vi "LockinDAQ.Write AO.vi"(8 "error in (no error)":errorcluster, 10 "AO []":waveform(dbl)[](array[waveform]), 11 "LockinDAQ":refnum<class "LockinDAQ.lvclass">) -> (0 "error out":errorcluster, 1 "AO":u32, 3 "LockinDAQ out":refnum<class "LockinDAQ.lvclass">)   [LabVIEW 2016, in "LockinDAQ.lvclass"]
uses:
  LockinDAQ.lvclass
  LockinDAQ.lvclass/LockinDAQ.ctl
  <vilib>/DAQmx/write.llb/DAQmx Write (Analog 1D Wfm NChan NSamp).vi
  <vilib>/DAQmx/miscellaneous.llb/DAQmx Fill In Error Info.vi
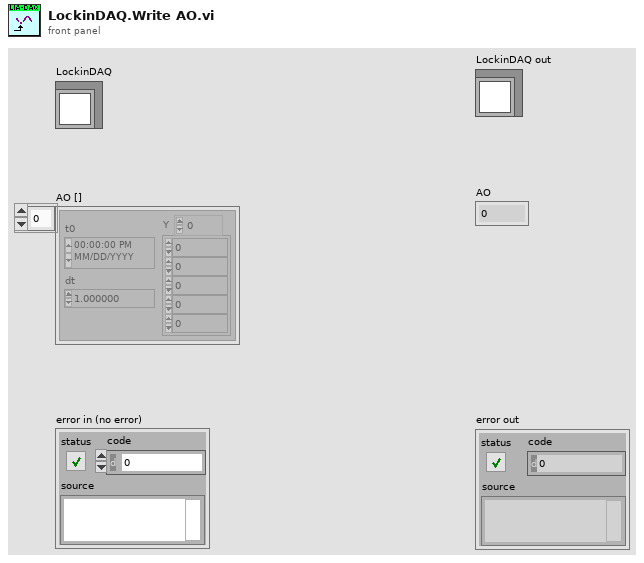
[diagram p1: front panel]
types:
  T1 = typedef "LockinDAQ.lvclass/DAQType-enum.ctl" = enum16{"None", "USB 4431", "PXI 446x"}
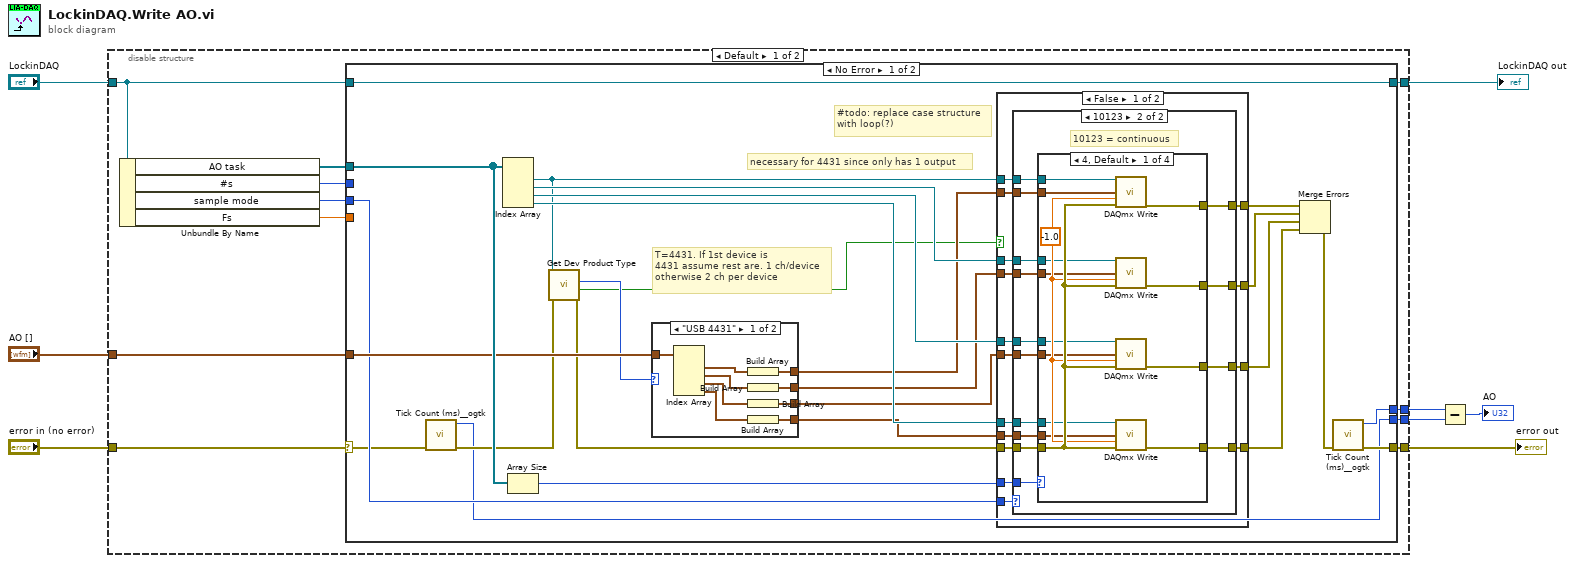
[diagram p0: block diagram]
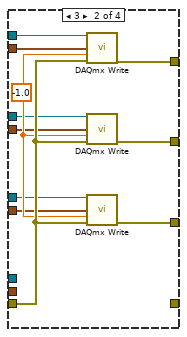
[diagram p3: hidden frame]
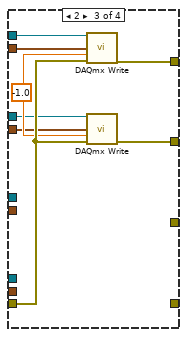
[diagram p4: hidden frame]
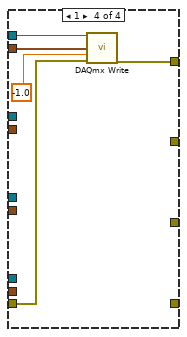
[diagram p5: hidden frame]
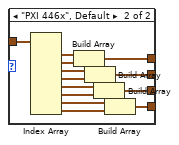
[diagram p7: hidden frame]
diagram:
  n1 = disable-structure shown="Default" {
    disable-tunnel: [w17 w140] -> w3
    disable-tunnel: "LockinDAQ" -> [w15 _]
    disable-tunnel: "AO []" -> [w16 w139]
    disable-tunnel: "error in (no error)" -> [w9 w140]
    disable-tunnel: [w14 _] -> w2
    disable-tunnel: [w13 _] -> w7
    disable-tunnel: [w12 _] -> w6
    frame condition #0 (active) {
      n2 = Unbundle By Name(w15) -> ("AO task"=w10:refnum<k21>[], "#s"=w19:i32, "sample mode"=w18:i32, "Fs"=w11:dbl)
      n3 = case shown="No Error" w9 {
        selector: w9 -> [w24 w137]
        tunnel: w19 -> [_ _]
        tunnel: w18 -> [w25 _]
        tunnel: [w42 w137] -> w17
        tunnel: w16 -> [w44 _]
        tunnel: w10 -> [w45 _]
        tunnel: w15 -> [w27 w138]
        tunnel: [w27 w138] -> w14
        tunnel: [w41 _] -> w13
        tunnel: [w20 _] -> w12
        tunnel: w11 -> [_ _]
        frame No Error {
          # "#todo: replace case structure\nwith loop(?)"
          # "T=4431. If 1st device is \n4431 assume rest are. 1 ch/device\notherwise 2 ch per device"
          # "necessary for 4431 since only has 1 output"
          n4 = call <userlib>:"Tick Count (ms)__ogtk.vi"("error in (no error)"=w24) -> ("error out"=w22:errorcluster, "millisecond timer value"=w20:u32)  [unwired: 9 in]
          n5 = Index Array(array=w45) -> (element #1=w36:refnum<k21>, element #2=w40:refnum<k21>, element #3=w39:refnum<k21>, element #4=w38:refnum<k21>)  [unwired: 4 in]
          n6 = Array Size(array=w45) -> (size(s)=w37:i32)
          n7 = call "Get Dev Product Type.vi"("error in (no error)"=w22, "Refnum in"=w36) -> ("error out"=w21:errorcluster, "DevIsSimulated"=w23:bool, "DAQ Type"=w31:T1)  [unwired: 6 in, 1 out]
          n8 = case shown="\"USB 4431\"" w31 {
            tunnel: [w123 w129] -> w33
            tunnel: [w122 w128] -> w34
            tunnel: [w121 w127] -> w35
            tunnel: [w119 w125] -> w32
            tunnel: w44 -> [w118 w124]
            frame "USB 4431" {
              n9 = Index Array(array=w118) -> (element #1=w120:waveform(dbl), element #2=w117:waveform(dbl), element #3=w116:waveform(dbl), element #4=w115:waveform(dbl))  [unwired: 4 in]
              n10 = Build Array(w120) -> (w119:waveform(dbl)[])
              n11 = Build Array(w117) -> (w123:waveform(dbl)[])
              n12 = Build Array(w116) -> (w122:waveform(dbl)[])
              n13 = Build Array(w115) -> (w121:waveform(dbl)[])
            }
            frame "PXI 446x", Default {
              n14 = Index Array(array=w124) -> (element #1=w126:waveform(dbl), element #2=w136:waveform(dbl), element #3=w135:waveform(dbl), element #4=w134:waveform(dbl), element #5=w133:waveform(dbl), element #6=w132:waveform(dbl), element #7=w131:waveform(dbl), element #8=w130:waveform(dbl))  [unwired: 8 in]
              n15 = Build Array(w126, w136) -> (w125:waveform(dbl)[])
              n16 = Build Array(w135, w134) -> (w129:waveform(dbl)[])
              n17 = Build Array(w133, w132) -> (w128:waveform(dbl)[])
              n18 = Build Array(w131, w130) -> (w127:waveform(dbl)[])
            }
          }
          n19 = case shown="False" w23 {
            tunnel: w40 -> [w60 _]
            tunnel: w39 -> [w59 _]
            tunnel: w38 -> [w58 _]
            tunnel: w37 -> [w57 _]
            tunnel: w36 -> [w56 _]
            tunnel: w35 -> [w55 _]
            tunnel: w34 -> [w54 _]
            tunnel: w33 -> [w53 _]
            tunnel: w32 -> [w52 _]
            tunnel: w21 -> [w51 w114]
            tunnel: [w50 _] -> w30
            tunnel: [w49 _] -> w29
            tunnel: [w48 w114] -> w28
            tunnel: [w46 _] -> w26
            tunnel: w25 -> [w47 _]
            frame False {
              n20 = case shown="10123" w47 {
                tunnel: w60 -> [_ w75]
                tunnel: w59 -> [_ w74]
                tunnel: w58 -> [_ w73]
                tunnel: [w61 w72] -> w48
                tunnel: [_ w71] -> w49
                tunnel: [_ w70] -> w50
                tunnel: [_ w69] -> w46
                tunnel: w57 -> [_ w68]
                tunnel: w56 -> [_ w67]
                tunnel: w55 -> [_ w66]
                tunnel: w54 -> [_ w65]
                tunnel: w53 -> [_ w64]
                tunnel: w52 -> [_ w63]
                tunnel: w51 -> [w61 w62]
                frame 10178, Default {
                  # "10178 = finite sample mode (IV\nmode). Do not try to write\nmore samples to the buffer"
                }
                frame 10123 {
                  # "10123 = continuous"
                  n21 = case shown="4, Default" w68 {
                    tunnel: w62 -> [w89 w100 w108 w113]
                    tunnel: w75 -> [w87 w98 w106 _]
                    tunnel: w74 -> [w86 w97 _ _]
                    tunnel: w73 -> [w85 _ _ _]
                    tunnel: w64 -> [w84 w96 w105 _]
                    tunnel: w65 -> [w83 w95 _ _]
                    tunnel: w66 -> [w82 _ _ _]
                    tunnel: [w81 w94 w104 w111] -> w72
                    tunnel: [w80 w93 w103 _] -> w71
                    tunnel: [w79 w92 _ _] -> w70
                    tunnel: [w78 _ _ _] -> w69
                    tunnel: w67 -> [w77 w91 w102 w110]
                    tunnel: w63 -> [w76 w90 w101 w109]
                    frame 4, Default {
                      w88 = -1.0 ("timeout")
                      n22 = call-poly <vilib>:"DAQmx Write.vi"("task/channels in"=w77, "data"=w76, "timeout"=w88, "error in"=w89) -> ("error out"=w81:errorcluster)  [unwired: 9 in, 2 out]
                      n23 = call-poly <vilib>:"DAQmx Write.vi"("task/channels in"=w87, "data"=w84, "timeout"=w88, "error in"=w89) -> ("error out"=w80:errorcluster)  [unwired: 9 in, 2 out]
                      n24 = call-poly <vilib>:"DAQmx Write.vi"("task/channels in"=w86, "data"=w83, "timeout"=w88, "error in"=w89) -> ("error out"=w79:errorcluster)  [unwired: 9 in, 2 out]
                      n25 = call-poly <vilib>:"DAQmx Write.vi"("task/channels in"=w85, "data"=w82, "timeout"=w88, "error in"=w89) -> ("error out"=w78:errorcluster)  [unwired: 9 in, 2 out]
                    }
                    frame 3 {
                      w99 = -1.0 ("timeout")
                      n26 = call-poly <vilib>:"DAQmx Write.vi"("task/channels in"=w91, "data"=w90, "timeout"=w99, "error in"=w100) -> ("error out"=w94:errorcluster)  [unwired: 9 in, 2 out]
                      n27 = call-poly <vilib>:"DAQmx Write.vi"("task/channels in"=w98, "data"=w96, "timeout"=w99, "error in"=w100) -> ("error out"=w93:errorcluster)  [unwired: 9 in, 2 out]
                      n28 = call-poly <vilib>:"DAQmx Write.vi"("task/channels in"=w97, "data"=w95, "timeout"=w99, "error in"=w100) -> ("error out"=w92:errorcluster)  [unwired: 9 in, 2 out]
                    }
                    frame 2 {
                      w107 = -1.0 ("timeout")
                      n29 = call-poly <vilib>:"DAQmx Write.vi"("task/channels in"=w102, "data"=w101, "timeout"=w107, "error in"=w108) -> ("error out"=w104:errorcluster)  [unwired: 9 in, 2 out]
                      n30 = call-poly <vilib>:"DAQmx Write.vi"("task/channels in"=w106, "data"=w105, "timeout"=w107, "error in"=w108) -> ("error out"=w103:errorcluster)  [unwired: 9 in, 2 out]
                    }
                    frame 1 {
                      n31 = call-poly <vilib>:"DAQmx Write.vi"("task/channels in"=w110, "data"=w109, "timeout"=-1.0, "error in"=w113) -> ("error out"=w111:errorcluster)  [unwired: 9 in, 2 out]
                    }
                  }
                }
              }
            }
            frame True {
            }
          }
          n32 = Merge Errors(w28, w29, w30, w26) -> (w43:errorcluster)
          n33 = call <userlib>:"Tick Count (ms)__ogtk.vi"("error in (no error)"=w43) -> ("error out"=w42:errorcluster, "millisecond timer value"=w41:u32)  [unwired: 9 in]
        }
        frame Error {
        }
      }
    }
    frame condition #1 {
    }
  }
  "error out" <- w3
  "LockinDAQ out" <- w2
  n34 = Subtract(x=w7, y=w6) -> (x-y=→"AO":u32)
